vi "sv_Search with Tolerance for Element in Array (DBL).vi"(6 "tolerance":dbl=0.0001, 9 "start index":i32, 10 "element":dbl format="%.4g", 11 "1D array":dbl[](array[numeric]) format="%.4g") -> (1 "found index":i32, 2 "found element":dbl, 3 "found?":bool)   [LabVIEW 2017]
doc: "Use this VI to search for numeric elements within a 1D array of DBL. \n\nThis VI cannot be used to search for special values: Inf, -Inf, NaN. This VI can find numeric elements within an array containing special values: Inf, -Inf, NaN."
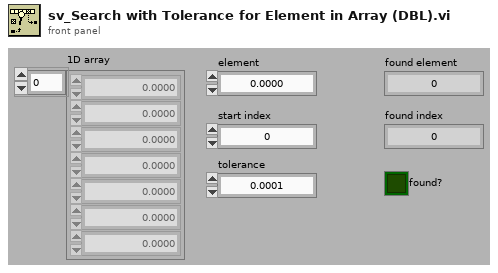
[diagram p1: front panel]
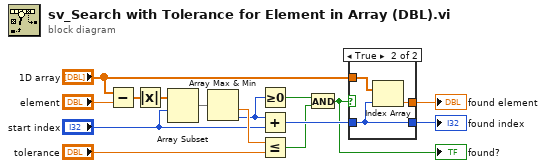
[diagram p0: block diagram]
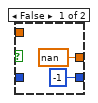
[diagram p2: hidden frame]
diagram:
  n1 = Subtract(x="1D array", y="element") -> (x-y=w14:dbl[])
  n2 = Absolute Value(x=w14) -> (abs(x)=w8:dbl[])
  n3 = Array Subset(array=w8, index="start index") -> (w7:dbl[])  [unwired: 1 in]
  n4 = Array Max & Min(array=w7) -> (min value=w13:dbl, min index (indices)=w4:i32)  [unwired: 2 out]
  n5 = Greater Or Equal To 0?(x=w4) -> (x >= 0?=w3:bool)
  n6 = Add(x=w4, y="start index") -> (x+y=w5:i32)
  n7 = Less Or Equal?(x=w13, y="tolerance") -> (x <= y?=w2:bool)
  n8 = And(x=w3, y=w2) -> (x .and. y?=w1:bool)
  "found?" <- w1
  n9 = case shown="True" w1 {
    tunnel: "1D array" -> [_ w20]
    tunnel: w5 -> [_ w18]
    tunnel: [nan ("Numeric") w19] -> w11
    tunnel: [-1 w18] -> w9
    frame False {
    }
    frame True {
      n10 = Index Array(array=w20, index=w18) -> (element=w19:dbl)
    }
  }
  "found element" <- w11
  "found index" <- w9
